vi "RxBfrPkt - Add Packet.vi"(8 "error in (no error)":errorcluster, 9 "New Packet ID":i32, 10 "New Packet Name":string, 11 "Item Ref in":T1=18446744073709551615 format="%.0x") -> (0 "error out":errorcluster, 2 "New Packet Ref":T1=18446744073709551615 format="%.0x", 3 "Item Ref Out":T1=18446744073709551615 format="%.0x")   [LabVIEW 2019, in "UDP-Custom-Device System Explorer.lvlib"]
uses:
  UDP-Custom-Device System Explorer.lvlib
  <vilib>/NI VeriStand/Custom Device API/Custom Device Item Ref.ctl
  Shared/Constants.vi
  Property Accessors/Shared Section Accessors.lvlib
  <vilib>/NI VeriStand/Custom Device API/Custom Device API.lvlib
  Property Accessors/Shared Packet Accessors.lvlib
  Shared/UDP-Custom-Device Shared.lvlib
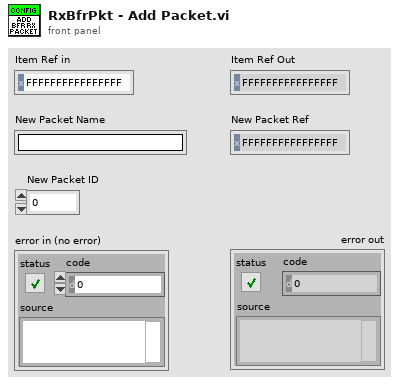
[diagram p1: front panel]
types:
  T1 = typedef "Custom Device API.lvlib/Custom Device Item Ref.ctl" = u64
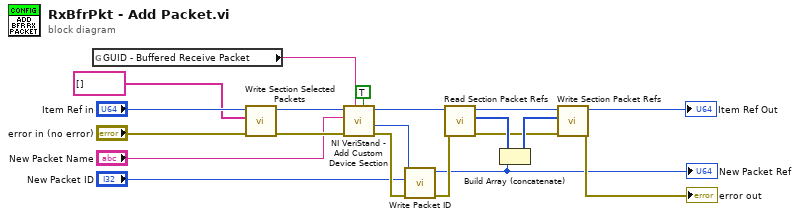
[diagram p0: block diagram]
diagram:
  n1 = global read "Constants.vi" "GUID - Buffered Receive Packet"() -> (w3:string)
  n2 = call "Write Section Selected Packets.vi"("error in (no error)"="error in (no error)", "Selected Packets"=string[] [] ("Value"), "Node Ptr"="Item Ref in") -> ("error out"=w12:errorcluster, "Node Ptr out"=w11:T1)  [unwired: 7 in]
  n3 = call <vilib>:"NI VeriStand - Add Custom Device Section.vi"("Highlight? (F)"=TRUE, "GUID (Default Section)"=w3, "error in (no error)"=w12, "Section Name"="New Packet Name", "Parent Ref in"=w11) -> ("error out"=w20:errorcluster, "Section Ptr"=w19:T1, "Parent Ref out"=w18:T1)  [unwired: 3 in, 1 out]
  n4 = call "Write Packet ID.vi"("error in (no error)"=w20, "Packet ID"="New Packet ID", "Node Ptr"=w19) -> ("error out"=w13:errorcluster, "Node Ptr out"=w1:T1)  [unwired: 7 in]
  "New Packet Ref" <- w1
  n5 = call "Read Section Packet Refs.vi"("error in (no error)"=w13, "Node Ptr"=w18) -> ("error out"=w14:errorcluster, "Dependent Node Refs"=w16:T1[], "Node Ptr out"=w17:T1)  [unwired: 7 in]
  n6 = Build Array (concatenate)(w16, w1) -> (w15:T1[])
  n7 = call "Write Section Packet Refs.vi"("error in (no error)"=w14, "Dependent Node Refs"=w15, "Node Ptr"=w17) -> ("error out"=→"error out":errorcluster, "Node Ptr out"=→"Item Ref Out":T1)  [unwired: 7 in]
